vi "aft_ANC_State Machine.vi"(7 "filter length":u32, 10 "initialize x read address":u32, 11 "index":i32) -> (0 "x read address":u32, 1 "coefficient read address":u32, 2 "coefficient write enable":bool, 3 "coefficient write address":u32, 4 "stop":bool)   [LabVIEW 2019]
doc: "This VI generates addresses for reading and writing RAM.\n\nThis VI is an instance VI. Complete the following steps to convert this instance VI into a subVI.\n\n(1) Right-click the instance VI.\n(2) Select <b>Open Front Panel</b> from the shortcut menu.\n(3) Save the VI."
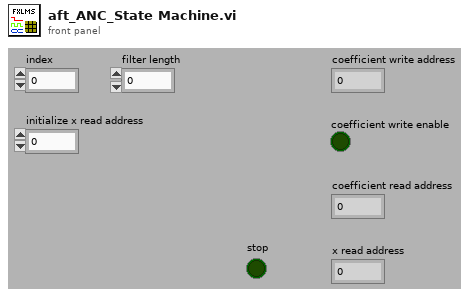
[diagram p1: front panel]
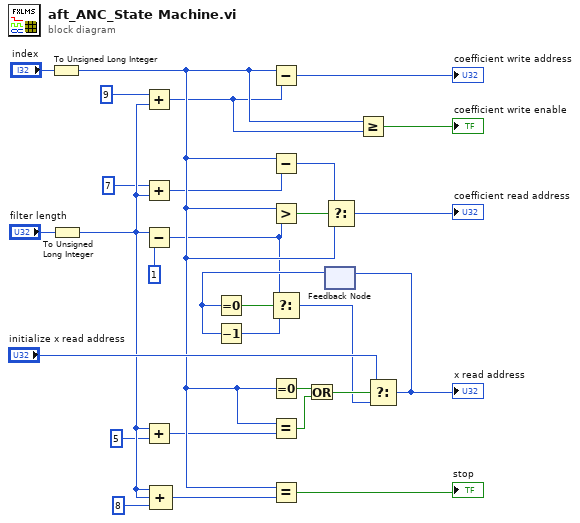
[diagram p0: block diagram]
diagram:
  n1 = To Unsigned Long Integer(number="index") -> (unsigned 32bit integer=w21:u32)
  n2 = To Unsigned Long Integer(number="filter length") -> (unsigned 32bit integer=w23:u32)
  n3 = Add(x=u32 9, y=w23) -> (x+y=w3:u32)
  n4 = Add(x=u32 7, y=w23) -> (x+y=w8:u32)
  n5 = Subtract(x=w23, y=u32 1) -> (x-y=w6:u32)
  n6 = Add(x=w23, y=u32 5) -> (x+y=w4:u32)
  n7 = Compound Arithmetic op=ADD(w23, w23, u32 8 ("value")) -> (w2:u32)
  n8 = Subtract(x=w21, y=w3) -> (x-y=→"coefficient write address":u32)
  n9 = Subtract(x=w21, y=w8) -> (x-y=w18:u32)
  n10 = Greater?(x=w21, y=w6) -> (0:w19:bool)
  n11 = Equal To 0?(x=w21) -> (x = 0?=w11:bool)
  n12 = Equal?(x=w21, y=w4) -> (x = y?=w17:bool)
  n13 = Equal?(x=w21, y=w2) -> (x = y?=→"stop":bool)
  n14 = Or(x=w11, y=w17) -> (x .or. y?=w16:bool)
  n15 = feedback #1() -> (w12:u32)  [unwired: 1 out]
  n16 = Equal To 0?(x=w12) -> (x = 0?=w15:bool)
  n17 = Decrement(x=w12) -> (x-1=w14:u32)
  n18 = Select(t=w6, s=w15, f=w14) -> (s? t:f=w13:u32)
  n19 = Select(t=w18, s=w19, f=w21) -> (s? t:f=→"coefficient read address":u32)
  n20 = Greater Or Equal?(x=w21, y=w3) -> (x >= y?=→"coefficient write enable":bool)
  n21 = Select(t="initialize x read address", s=w16, f=w13) -> (s? t:f=w27:u32)
  "x read address" <- w27
  n22 = feedback-in #1(w27) -> ()
